vi "Queue Self Alias.vi"(11 "jettl Event Actor in":refnum<class "jettl Event Actor.lvclass">) -> (2 "Queue Self Alias":string)   [LabVIEW 2021, in "jettl.lvlib" / "jettl Event Actor.lvclass"]
uses:
  jettl Event Actor.lvclass
  jettl Event Actor.lvclass/jettl Event Actor.ctl
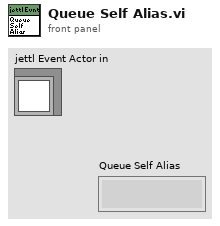
[diagram p1: front panel]
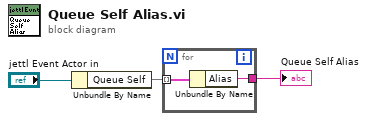
[diagram p0: block diagram]
diagram:
  n1 = Unbundle By Name("jettl Event Actor in") -> ("Queue Self"=w3:map{string, refnum<data-value>})
  n2 = for {
    tunnel: w3 -> [w5] mode=indexing
    tunnel: [w4] -> w2
    n3 = Unbundle By Name(w5) -> ("Alias"=w4:string)
  }
  "Queue Self Alias" <- w2
